vi "Init - Node Config Pop Up.vi"(8 "error in (no error)":errorcluster) -> (0 "error out":errorcluster, 1 "Configuration Files Path Out":path, 2 "Node_ID Out":u16)   [LabVIEW 2016, in "PXImc Custom Device System Explorer.lvlib"]
uses:
  PXImc Custom Device System Explorer.lvlib
panel:
  in  "OK":bool
  in  "Node_ID":u16
  in  "Configuration Files Path":path
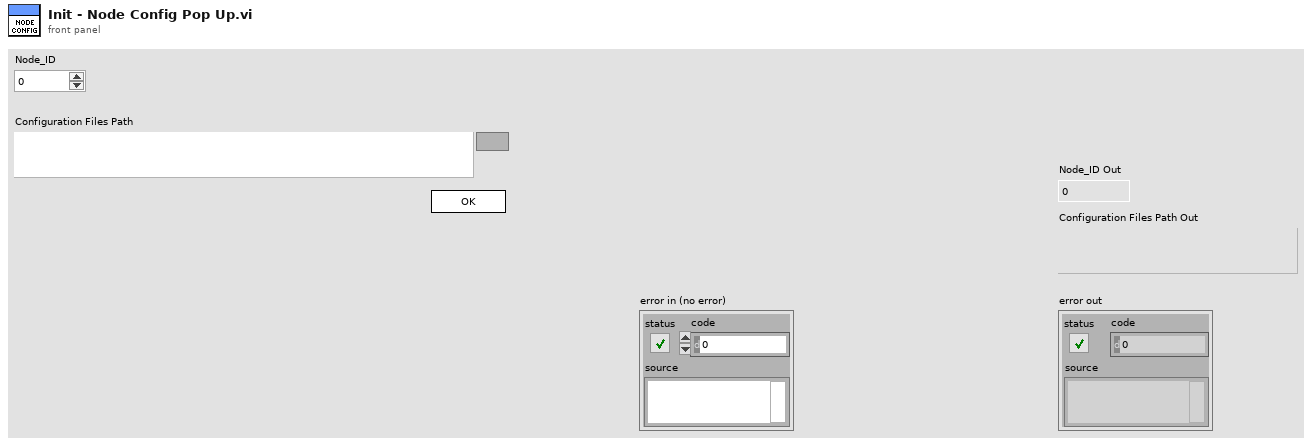
[diagram p1: front panel]
types:
  T1 = enum8{"Enabled", "Disabled", "Disabled and Grayed Out"}
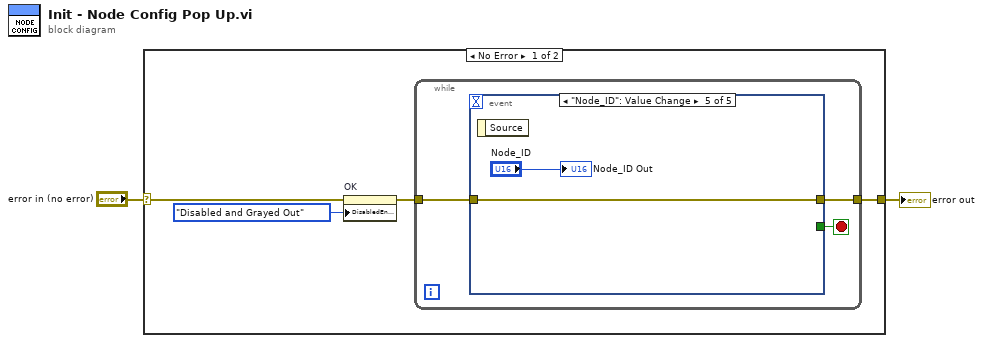
[diagram p0: block diagram]
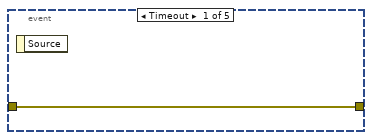
[diagram p2: hidden frame]
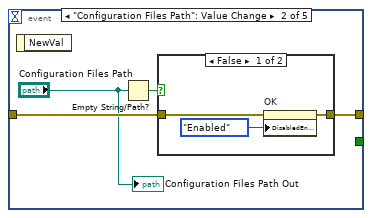
[diagram p3: hidden frame]
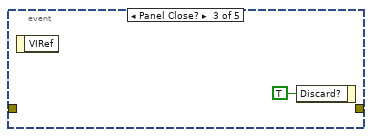
[diagram p5: hidden frame]
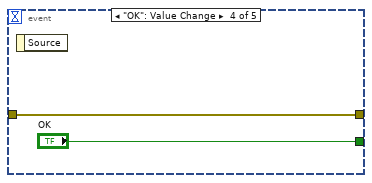
[diagram p6: hidden frame]
diagram:
  n1 = case shown="No Error" "error in (no error)" {
    selector: "error in (no error)" -> [w6 w24]
    tunnel: [w3 w24] -> w1
    frame No Error {
      n2 = property on="OK" class="Bool"(error in=w6, "DisabledEnum"=T1."Disabled and Grayed Out" ("Disabled")) -> (error out=w4:errorcluster)  [unwired: 1 in, 1 out]
      n3 = while {
        tunnel: w4 -> [w9]
        tunnel: [w8] -> w3
        stop <- w7 stop-if-true
        n4 = event shown="[4] \"Node_ID\": Value Change" {
          selector: _ -> [_ _ _ _ _]
          dyn-events: _ -> [_ _ _ _ _]
          timeout: _ -> [_ _ _ _ _]
          tunnel: w9 -> [w10 w13 _ w20 w23]
          tunnel: [w10 w12 _ w20 w23] -> w8
          tunnel: [_ _ _ "OK" _] -> w7
          event Timeout {
            n5 = event-data() -> ()  [unwired: 1 in, 1 out]
          }
          event "Configuration Files Path": Value Change {
            n6 = event-data() -> ()  [unwired: 1 in, 1 out]
            n7 = Empty String/Path?(string/path="Configuration Files Path") -> (empty?=w14:bool)
            n8 = case shown="False" w14 {
              tunnel: w13 -> [w16 w18]
              tunnel: [w15 w18] -> w12
              frame False {
                n9 = property on="OK" class="Bool"(error in=w16, "DisabledEnum"=T1."Enabled" ("Disabled")) -> (error out=w15:errorcluster)  [unwired: 1 in, 1 out]
              }
              frame True {
              }
            }
            "Configuration Files Path Out" <- "Configuration Files Path"
          }
          event Panel Close? {
            n10 = event-data() -> ()  [unwired: 1 in, 1 out]
            n11 = event-data("Discard?"=TRUE) -> ()  [unwired: 1 in, 1 out]
          }
          event "OK": Value Change {
            n12 = event-data() -> ()  [unwired: 1 in, 1 out]
          }
          event "Node_ID": Value Change {
            n13 = event-data() -> ()  [unwired: 1 in, 1 out]
            "Node_ID Out" <- "Node_ID"
          }
        }
      }
    }
    frame Error {
    }
  }
  "error out" <- w1
